vi "Calibration proud.vi"(5 "linearni":dbl, 6 "absolutni":dbl, 7 "kvadraticky":dbl, 8 "error in (no error)":errorcluster, 9 "Rozsah":string(combo), 10 "Combo Box":string(combo), 11 "VISA resource name":refnum<visa-resource-name>) -> (0 "error out":errorcluster, 3 "VISA resource name out":refnum<visa-resource-name>)   [LabVIEW 2024, in "EFmeter.lvlib"]
uses:
  <instrlib>/EFmeter/EFmeter.lvlib
panel:
  out "Error Message":string
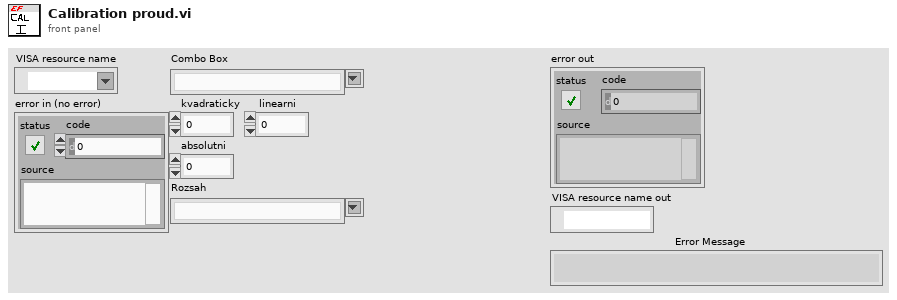
[diagram p1: front panel]
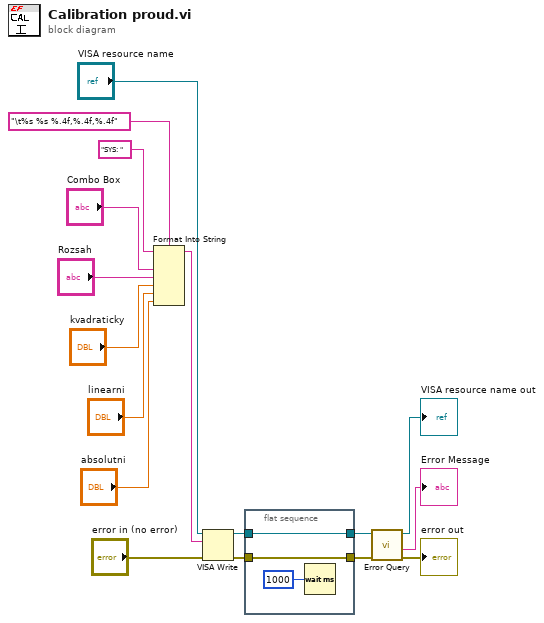
[diagram p0: block diagram]
diagram:
  n1 = Format Into String(format string="\t%s %s %.4f,%.4f,%.4f", initial string="SYS: ", "Combo Box", "Rozsah", "kvadraticky", "linearni", "absolutni") -> (resulting string=w13:string)  [unwired: 1 in, 1 out]
  n2 = VISA Write(VISA resource name="VISA resource name", write buffer=w13, error in (no error)="error in (no error)") -> (VISA resource name out=w12:refnum<visa-resource-name>, error out=w11:errorcluster)  [unwired: 1 out]
  n3 = flat-sequence {
    tunnel: w12 -> [w20]
    tunnel: [w20] -> w9
    tunnel: [w19] -> w10
    tunnel: w11 -> [w19]
    frame #0 {
      n4 = Wait (ms)(milliseconds to wait=u32 1000) -> ()  [unwired: 1 out]
    }
  }
  n5 = call <instrlib>:"Error Query.vi"("error in (no error)"=w10, "VISA resource name"=w9) -> ("error out"=→"error out":errorcluster, "Error Message"=→"Error Message":string, "VISA resource name out"=→"VISA resource name out":refnum<visa-resource-name>)  [unwired: 6 in, 1 out]
